vi "merge_channels.vi"(6 "FIFO_3":u16[](array[numeric]), 7 "number of channels":i32, 8 "error in (no error)":errorcluster, 9 "FIFO_2":u16[](array[numeric]), 10 "FIFO_1":u16[](array[numeric]), 11 "DL090211FPGAWrapper in":refnum<class "FPGAWrapperDL090211Galvo.lvclass">) -> (0 "error out":errorcluster, 2 "channels raw data block":T1, 3 "DL090211FPGAWrapper out":refnum<class "FPGAWrapperDL090211Galvo.lvclass">)   [LabVIEW 2010, in "FPGAWrapperDL090211Galvo.lvclass"]
uses:
  FPGAWrapperDL090211Galvo.lvclass
  common/arrays/pixel_raw_data_array.ctl
  FPGAWrapperDL090211Galvo.lvclass/FPGAWrapperDL090211Galvo.ctl
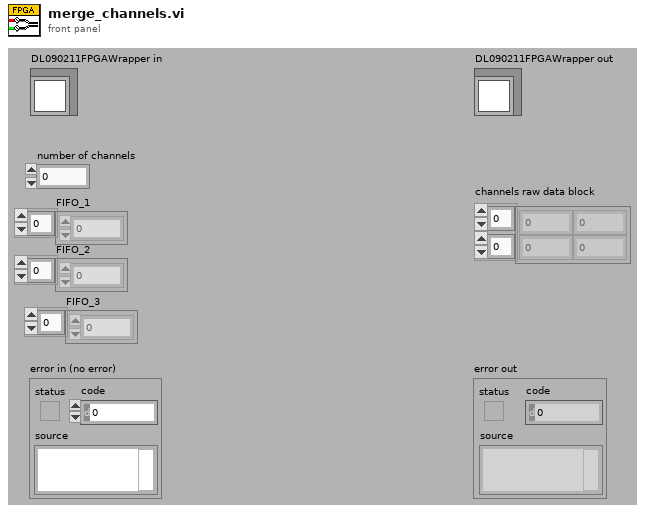
[diagram p1: front panel]
types:
  T1 = typedef "pixel_raw_data_array.ctl" = dbl[][]
  T2 = typedef "pixel_to_host_enum.ctl" = enum16{"3-channel mode", "4-channel mode"}
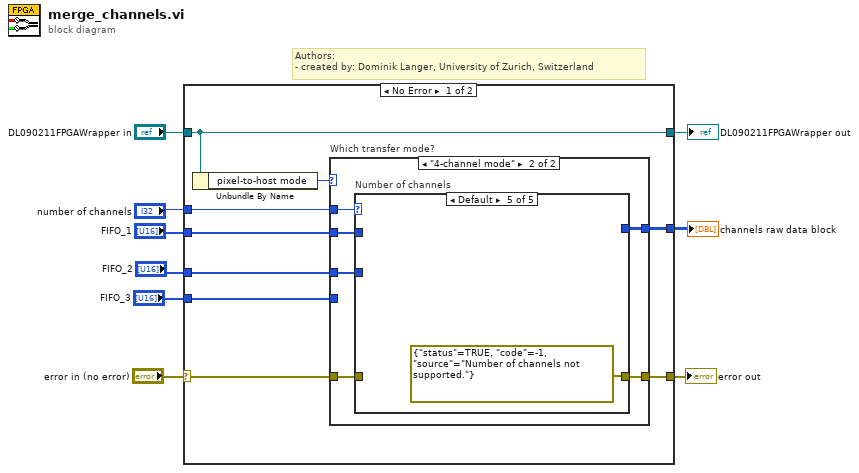
[diagram p0: block diagram]
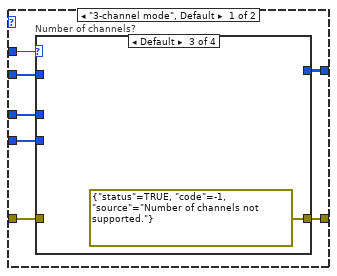
[diagram p2: hidden frame]
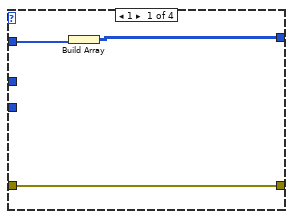
[diagram p3: hidden frame]
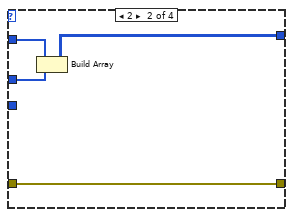
[diagram p4: hidden frame]
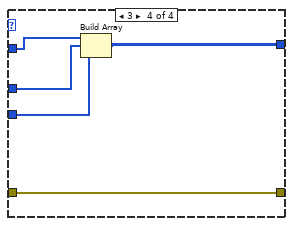
[diagram p5: hidden frame]
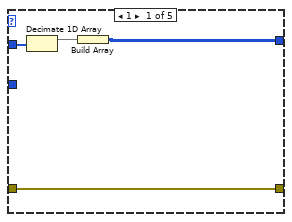
[diagram p6: hidden frame]
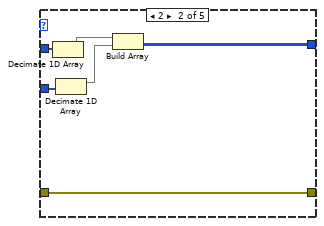
[diagram p7: hidden frame]
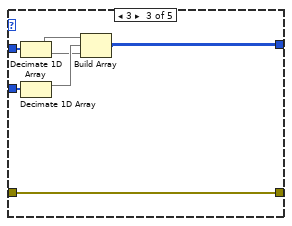
[diagram p8: hidden frame]
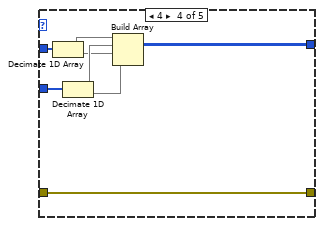
[diagram p9: hidden frame]
diagram:
  # "Authors: \n- created by: Dominik Langer, University of Zurich, Switzerland"
  n1 = case shown="No Error" "error in (no error)" {
    selector: "error in (no error)" -> [w13 w72]
    tunnel: [w12 w72] -> w8
    tunnel: [w11 w71] -> w6
    tunnel: "DL090211FPGAWrapper in" -> [w11 w71]
    tunnel: "number of channels" -> [w18 _]
    tunnel: "FIFO_1" -> [w17 _]
    tunnel: "FIFO_2" -> [w16 _]
    tunnel: [w15 _] -> w2
    tunnel: "FIFO_3" -> [w14 _]
    frame No Error {
      n2 = Unbundle By Name(w11) -> ("pixel-to-host mode"=w10:T2)
      n3 = case "Which transfer mode?" shown="\"4-channel mode\"" w10 {
        tunnel: w18 -> [w25 w44]
        tunnel: w17 -> [w24 w43]
        tunnel: w16 -> [w23 w42]
        tunnel: [w21 w41] -> w15
        tunnel: w14 -> [w22 _]
        tunnel: w13 -> [w20 w40]
        tunnel: [w19 w39] -> w12
        frame "3-channel mode", Default {
          n4 = case "Number of channels?" shown="Default" w25 {
            tunnel: w23 -> [_ w30 _ w36]
            tunnel: [w28 w32 _ w38] -> w21
            tunnel: w24 -> [w27 w31 _ w37]
            tunnel: w22 -> [_ _ _ w35]
            tunnel: w20 -> [w26 w29 _ w34]
            tunnel: [w26 w29 errorcluster {"status"=TRUE, "code"=-1, "source"="Number of channels not supported."} ("error IO") w34] -> w19
            frame 1 {
              n5 = Build Array(w27) -> (w28:u16[][])
            }
            frame 2 {
              n6 = Build Array(w31, w30) -> (w32:u16[][])
            }
            frame Default {
            }
            frame 3 {
              n7 = Build Array(w37, w36, w35) -> (w38:u16[][])
            }
          }
        }
        frame "4-channel mode" {
          n8 = case "Number of channels" shown="Default" w44 {
            tunnel: w42 -> [_ w51 w59 w69 _]
            tunnel: w43 -> [w47 w53 w60 w68 _]
            tunnel: [w48 w54 w61 w67 _] -> w41
            tunnel: w40 -> [w45 w49 w55 w62 _]
            tunnel: [w45 w49 w55 w62 errorcluster {"status"=TRUE, "code"=-1, "source"="Number of channels not supported."} ("error IO")] -> w39
            frame 1 {
              n9 = Decimate 1D Array(w47) -> (w46:u16[])  [unwired: 1 out]
              n10 = Build Array(w46) -> (w48:u16[][])
            }
            frame 2 {
              n11 = Decimate 1D Array(w53) -> (w52:u16[])  [unwired: 1 out]
              n12 = Decimate 1D Array(w51) -> (w50:u16[])  [unwired: 1 out]
              n13 = Build Array(w52, w50) -> (w54:u16[][])
            }
            frame 3 {
              n14 = Decimate 1D Array(w60) -> (w58:u16[], w56:u16[])
              n15 = Decimate 1D Array(w59) -> (w57:u16[])  [unwired: 1 out]
              n16 = Build Array(w58, w57, w56) -> (w61:u16[][])
            }
            frame 4 {
              n17 = Decimate 1D Array(w68) -> (w66:u16[], w63:u16[])
              n18 = Decimate 1D Array(w69) -> (w64:u16[], w65:u16[])
              n19 = Build Array(w66, w64, w63, w65) -> (w67:u16[][])
            }
            frame Default {
            }
          }
        }
      }
    }
    frame Error {
    }
  }
  "error out" <- w8
  "DL090211FPGAWrapper out" <- w6
  "channels raw data block" <- w2
